vi "ReadFlashTime.vi"(10 "枚举":enum16{"测充电灯亮灭", "测充电灯闪烁", "测大灯1和2亮灭", "测大灯闪烁"}(ring), 11 "TestIndex":i32) -> (2 "Value":u8)   [LabVIEW 2015]
uses:
  Global variable.vi
  <vilib>/Instr/_visa.llb/VISA Configure Serial Port (Instr).vi
panel:
  out "数值 2":i32
  out "字符串":string
  out "数值":i32
  out "数组":i32[](array[numeric])
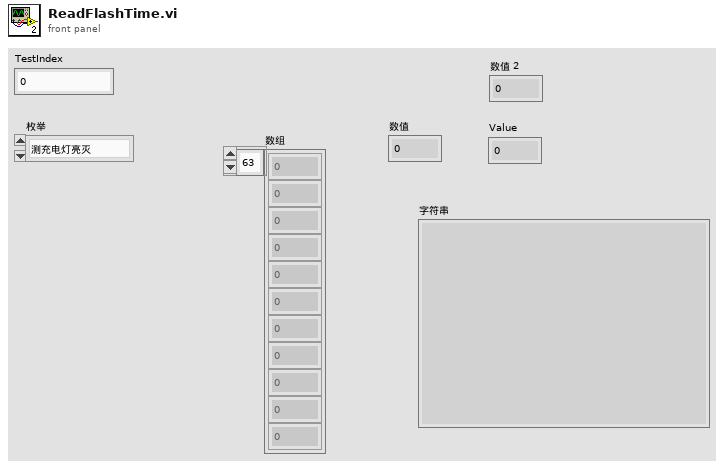
[diagram p1: front panel]
types:
  T1 = cluster{"CH1603":refnum<visa-resource-name>, "VSMD124_025T":refnum<visa-resource-name>, "RPM表":refnum<visa-resource-name>, "ACSource安姆泰克":refnum<visa-resource-name>, "VICTOR8246":refnum<visa-resource-name>, "MSP-Gang":refnum<visa-resource-name>, "6724Power":refnum<visa-resource-name>, "electric load":refnum<visa-resource-name>, "Arduino":refnum<visa-resource-name>, "6322Power":refnum<visa-resource-name>}
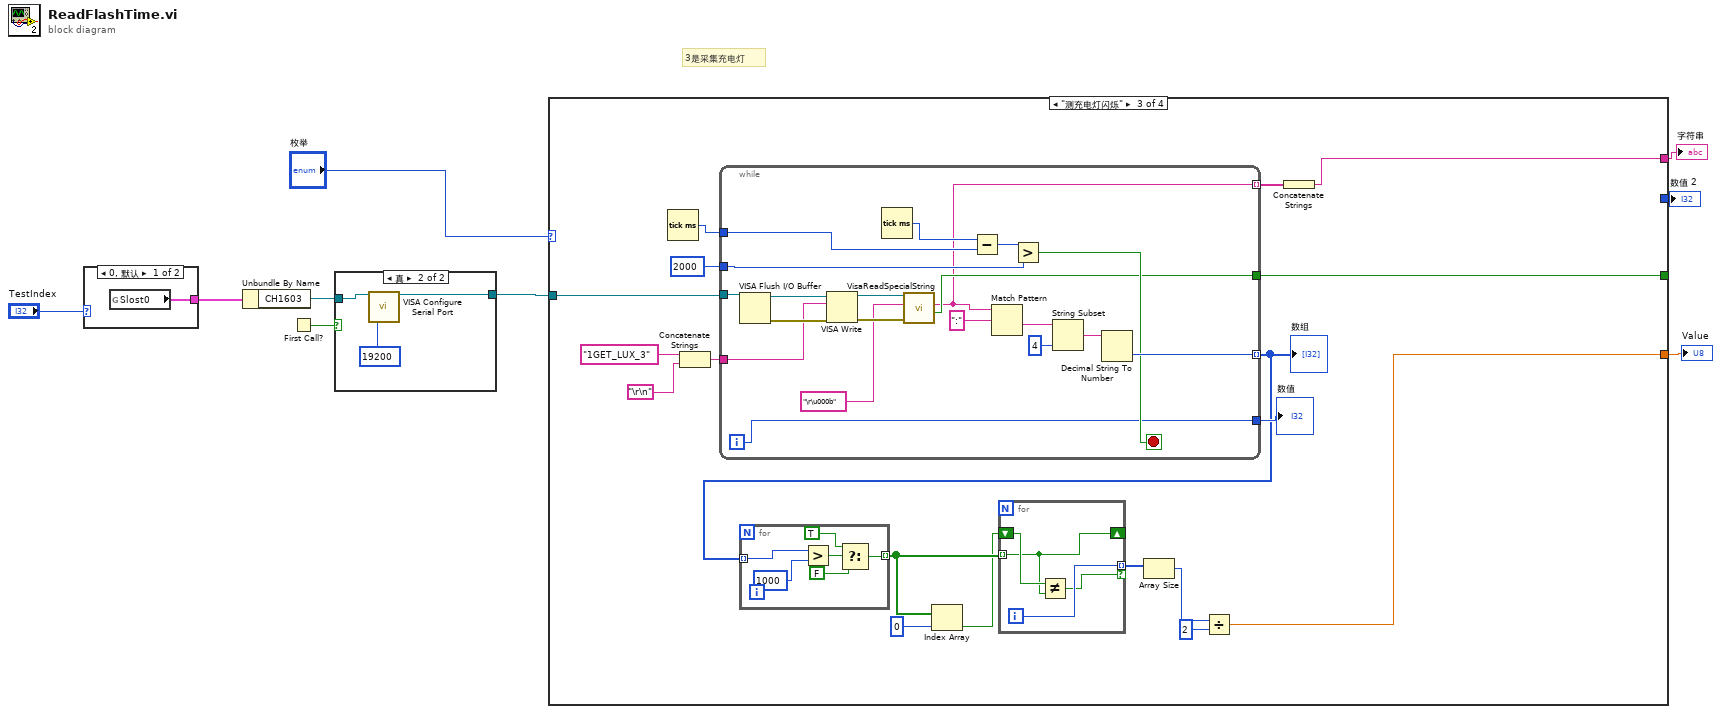
[diagram p0: block diagram]
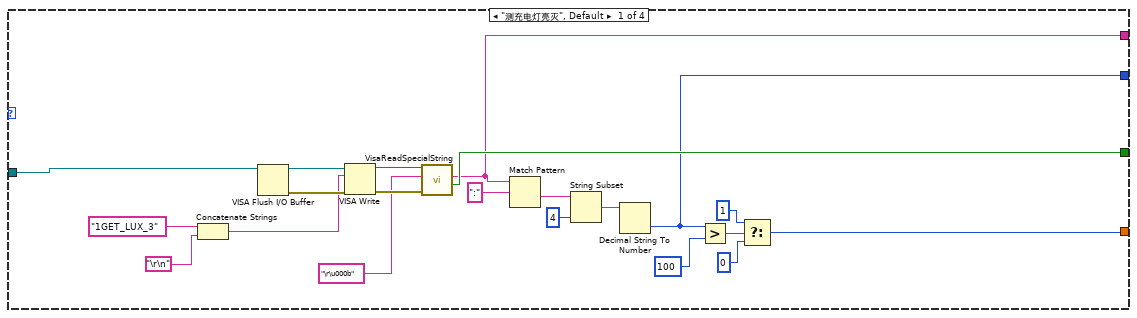
[diagram p3: hidden frame]
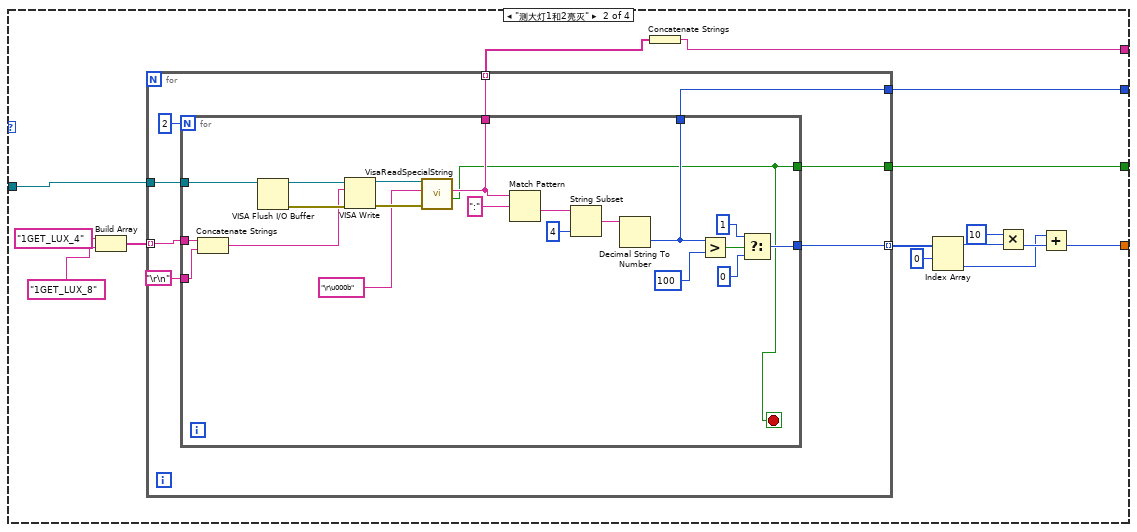
[diagram p4: hidden frame]
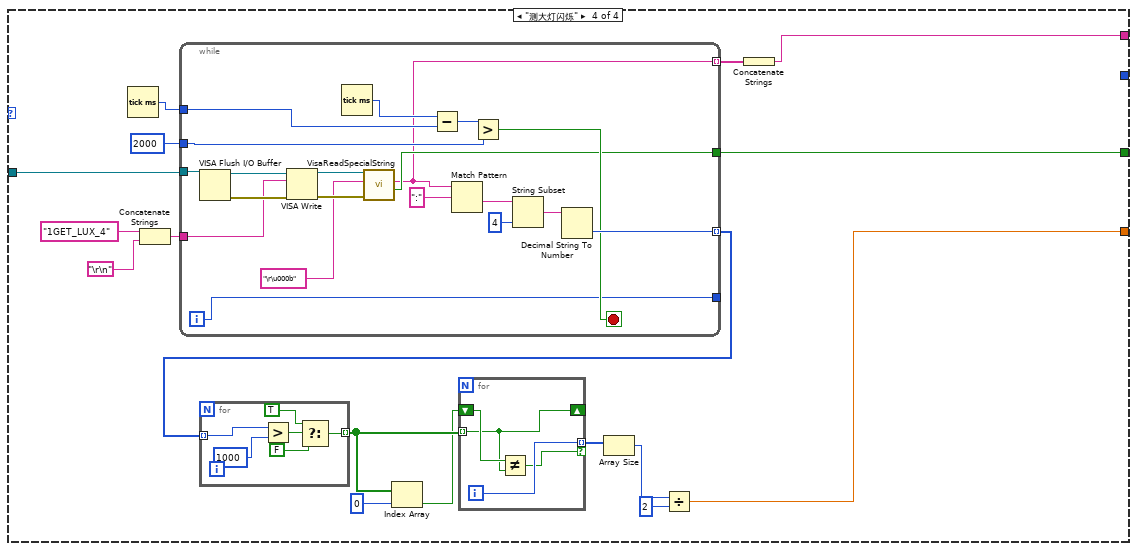
[diagram p5: hidden frame]
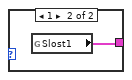
[diagram p6: hidden frame]
diagram:
  # "3是采集充电灯"
  n1 = case shown="0, 默认" "TestIndex" {
    tunnel: [w10 w11] -> w8
    frame 0, Default {
      n2 = global read "Global variable.vi" "Slost0"() -> (w10:T1)
    }
    frame 1 {
      n3 = global read "Global variable.vi" "Slost1"() -> (w11:T1)
    }
  }
  n4 = Unbundle By Name(w8) -> ("CH1603"=w5:refnum<visa-resource-name>)
  n5 = First Call?() -> (First Call?: T/F=w6:bool)
  n6 = case shown="真" w6 {
    tunnel: w5 -> [w12 w15]
    tunnel: [w12 w13] -> w4
    frame False {
    }
    frame True {
      n7 = call-poly "VISA Configure Serial Port"("VISA resource name"=w15, "baud rate (9600)"=u32 19200) -> ("VISA resource name out"=w13:refnum<visa-resource-name>)  [unwired: 12 in, 1 out]
    }
  }
  n8 = case shown="\"测充电灯闪烁\"" "枚举" {
    tunnel: w4 -> [w25 w50 w98 w145]
    tunnel: [w21 w49 w91 w139] -> _
    tunnel: [w18 w40 w81 w129] -> w3
    tunnel: [w17 w47 _ _] -> w1
    tunnel: [w16 w37 w89 w137] -> w2
    frame "测充电灯亮灭", Default {
      n9 = Concatenate Strings("1GET_LUX_3", "\r\n") -> (w24:string)
      n10 = VISA Flush I/O Buffer(VISA resource name=w25) -> (VISA resource name out=w34:refnum<visa-resource-name>, error out=w33:errorcluster)  [unwired: 2 in]
      n11 = VISA Write(VISA resource name=w34, write buffer=w24, error in (no error)=w33) -> (VISA resource name out=w32:refnum<visa-resource-name>, error out=w31:errorcluster)  [unwired: 1 out]
      n12 = call "VisaReadSpecialString.vi"("error in (no error)"=w31, "正则表达式"="\r\u000b", "VISA resource name out"=w32) -> ("布尔"=w21:bool, "字符串"=w16:string)  [unwired: 5 in, 2 out]
      n13 = Match Pattern(string=w16, regular expression=":" ("搜索字符串/字符(-)")) -> (after substring=w28:string)  [unwired: 1 in, 3 out]
      n14 = String Subset(string=w28, length (rest)=4 ("长度（剩余）")) -> (substring=w26:string)  [unwired: 1 in]
      n15 = Decimal String To Number(string=w26) -> (number=w17:i32)  [unwired: 2 in, 1 out]
      n16 = Greater?(x=w17, y=100) -> (0:w22:bool)
      n17 = Select(t=u8 1, s=w22, f=u8 0 ("t")) -> (s? t:f=w18:u8)
    }
    frame "测大灯1和2亮灭" {
      n18 = Build Array("1GET_LUX_4", "1GET_LUX_8") -> (w46:string[])
      n19 = for {
        tunnel: w50 -> [w58]
        tunnel: [w57] -> w49
        tunnel: [w56] -> w48 mode=indexing
        tunnel: [w55] -> w47
        tunnel: [w54] -> w38 mode=indexing
        tunnel: w46 -> [w52] mode=indexing
        n20 = for {
          N: 2 -> [_]
          tunnel: w52 -> [w80]
          tunnel: "\r\n" -> [w79]
          tunnel: w58 -> [w69]
          tunnel: [w60] -> w57
          tunnel: [w63] -> w56
          tunnel: [w62] -> w55
          tunnel: [w61] -> w54
          stop <- w60 stop-if-true
          n21 = Concatenate Strings(w80, w79) -> (w68:string)
          n22 = VISA Flush I/O Buffer(VISA resource name=w69) -> (VISA resource name out=w78:refnum<visa-resource-name>, error out=w77:errorcluster)  [unwired: 2 in]
          n23 = VISA Write(VISA resource name=w78, write buffer=w68, error in (no error)=w77) -> (VISA resource name out=w76:refnum<visa-resource-name>, error out=w75:errorcluster)  [unwired: 1 out]
          n24 = call "VisaReadSpecialString.vi"("error in (no error)"=w75, "正则表达式"="\r\u000b", "VISA resource name out"=w76) -> ("布尔"=w60:bool, "字符串"=w61:string)  [unwired: 5 in, 2 out]
          n25 = Match Pattern(string=w61, regular expression=":" ("搜索字符串/字符(-)")) -> (after substring=w72:string)  [unwired: 1 in, 3 out]
          n26 = String Subset(string=w72, length (rest)=4 ("长度（剩余）")) -> (substring=w70:string)  [unwired: 1 in]
          n27 = Decimal String To Number(string=w70) -> (number=w62:i32)  [unwired: 2 in, 1 out]
          n28 = Greater?(x=w62, y=100) -> (0:w66:bool)
          n29 = Select(t=u8 1, s=w66, f=u8 0 ("t")) -> (s? t:f=w63:u8)
        }
      }
      n30 = Concatenate Strings(w38) -> (w37:string)
      n31 = Index Array(array=w48, index #1=0 ("索引")) -> (element #1=w44:u8, element #2=w39:u8)  [unwired: 1 in]
      n32 = Multiply(x=u8 10, y=w44) -> (x*y=w42:u8)
      n33 = Add(x=w39, y=w42) -> (x+y=w40:u8)
    }
    frame "测充电灯闪烁" {
      n34 = Tick Count (ms)() -> (millisecond timer value=w94:u32)
      n35 = Concatenate Strings("1GET_LUX_3", "\r\n") -> (w95:string)
      n36 = while {
        tunnel: w98 -> [w128]
        tunnel: w95 -> [w125]
        tunnel: [w117] -> w88 mode=indexing
        tunnel: w94 -> [w115]
        tunnel: u32 2000 ("y") -> [w113]
        tunnel: [w111] -> w92
        tunnel: [w110] -> w91
        tunnel: [w109] -> w90 mode=indexing
        i -> [w111]
        stop <- w112 stop-if-true
        n37 = VISA Flush I/O Buffer(VISA resource name=w128) -> (VISA resource name out=w127:refnum<visa-resource-name>, error out=w126:errorcluster)  [unwired: 2 in]
        n38 = VISA Write(VISA resource name=w127, write buffer=w125, error in (no error)=w126) -> (VISA resource name out=w124:refnum<visa-resource-name>, error out=w123:errorcluster)  [unwired: 1 out]
        n39 = Tick Count (ms)() -> (millisecond timer value=w116:u32)
        n40 = call "VisaReadSpecialString.vi"("error in (no error)"=w123, "正则表达式"="\r\u000b", "VISA resource name out"=w124) -> ("布尔"=w110:bool, "字符串"=w109:string)  [unwired: 5 in, 2 out]
        n41 = Subtract(x=w116, y=w115) -> (x-y=w114:u32)
        n42 = Match Pattern(string=w109, regular expression=":" ("搜索字符串/字符(-)")) -> (after substring=w120:string)  [unwired: 1 in, 3 out]
        n43 = Greater?(x=w114, y=w113) -> (0:w112:bool)
        n44 = String Subset(string=w120, length (rest)=4 ("长度（剩余）")) -> (substring=w118:string)  [unwired: 1 in]
        n45 = Decimal String To Number(string=w118) -> (number=w117:i32)  [unwired: 2 in, 1 out]
      }
      "数组" <- w88
      "数值" <- w92
      n46 = for {
        tunnel: w88 -> [w108] mode=indexing
        tunnel: [w103] -> w87 mode=indexing
        n47 = Greater?(x=w108, y=1000) -> (0:w106:bool)
        n48 = Select(t=TRUE, s=w106, f=FALSE) -> (s? t:f=w103:bool)
      }
      n49 = Index Array(array=w87, index=0 ("索引")) -> (element=w85:bool)
      n50 = for {
        tunnel: w87 -> [w101] mode=indexing
        shift-right: [w101] -> _
        shift-left: w85 -> [w102]
        tunnel: [w100] -> w84 mode=indexing if=w99
        i -> [w100]
        n51 = Not Equal?(x=w102, y=w101) -> (x != y?=w99:bool)
      }
      n52 = Array Size(array=w84) -> (size(s)=w83:i32)
      n53 = Divide(x=w83, y=2) -> (x/y=w81:dbl)
      n54 = Concatenate Strings(w90) -> (w89:string)
    }
    frame "测大灯闪烁" {
      n55 = Tick Count (ms)() -> (millisecond timer value=w141:u32)
      n56 = Concatenate Strings("1GET_LUX_4", "\r\n") -> (w142:string)
      n57 = while {
        tunnel: w145 -> [w175]
        tunnel: w142 -> [w172]
        tunnel: [w164] -> w136 mode=indexing
        tunnel: w141 -> [w162]
        tunnel: u32 2000 ("y") -> [w160]
        tunnel: [w158] -> _
        tunnel: [w157] -> w139
        tunnel: [w156] -> w138 mode=indexing
        i -> [w158]
        stop <- w159 stop-if-true
        n58 = VISA Flush I/O Buffer(VISA resource name=w175) -> (VISA resource name out=w174:refnum<visa-resource-name>, error out=w173:errorcluster)  [unwired: 2 in]
        n59 = VISA Write(VISA resource name=w174, write buffer=w172, error in (no error)=w173) -> (VISA resource name out=w171:refnum<visa-resource-name>, error out=w170:errorcluster)  [unwired: 1 out]
        n60 = Tick Count (ms)() -> (millisecond timer value=w163:u32)
        n61 = call "VisaReadSpecialString.vi"("error in (no error)"=w170, "正则表达式"="\r\u000b", "VISA resource name out"=w171) -> ("布尔"=w157:bool, "字符串"=w156:string)  [unwired: 5 in, 2 out]
        n62 = Subtract(x=w163, y=w162) -> (x-y=w161:u32)
        n63 = Match Pattern(string=w156, regular expression=":" ("搜索字符串/字符(-)")) -> (after substring=w167:string)  [unwired: 1 in, 3 out]
        n64 = Greater?(x=w161, y=w160) -> (0:w159:bool)
        n65 = String Subset(string=w167, length (rest)=4 ("长度（剩余）")) -> (substring=w165:string)  [unwired: 1 in]
        n66 = Decimal String To Number(string=w165) -> (number=w164:i32)  [unwired: 2 in, 1 out]
      }
      n67 = for {
        tunnel: w136 -> [w155] mode=indexing
        tunnel: [w150] -> w135 mode=indexing
        n68 = Greater?(x=w155, y=1000) -> (0:w153:bool)
        n69 = Select(t=TRUE, s=w153, f=FALSE) -> (s? t:f=w150:bool)
      }
      n70 = Index Array(array=w135, index=0 ("索引")) -> (element=w133:bool)
      n71 = for {
        tunnel: w135 -> [w148] mode=indexing
        shift-right: [w148] -> _
        shift-left: w133 -> [w149]
        tunnel: [w147] -> w132 mode=indexing if=w146
        i -> [w147]
        n72 = Not Equal?(x=w149, y=w148) -> (x != y?=w146:bool)
      }
      n73 = Array Size(array=w132) -> (size(s)=w131:i32)
      n74 = Divide(x=w131, y=2) -> (x/y=w129:dbl)
      n75 = Concatenate Strings(w138) -> (w137:string)
    }
  }
  "Value" <- w3
  "字符串" <- w2
  "数值 2" <- w1
